vi "EOL NVH Outputs Controls Buffer 2.0.vi"(0 "Mode":T2, 1 "Motion Number":u16, 3 "Part Number":u16, 5 "NVH Outputs Control":T3[](array[typedef]), 7 "NVH Configuration":T1, 9 "NVH Outputs":bool[](array[boolean]), 11 "Serial Number In":string, 13 "ambient  temp (deg F)":dbl) -> (4 "NVH Outputs Out":bool[](array[boolean]), 6 "NVH Single Outputs":bool, 10 "Serial Number Out":string, 12 "NVH_PartNumber Out":u16, 14 "NVH_MotionNumber":u16, 15 "NVH All Outputs":bool[](array[boolean]))   [LabVIEW 2018]
uses:
  02.Type Def's/NVH Digital Output.ctl
  02.Type Def's/NVH Mode Control 2.0.ctl
  02.Type Def's/station nvh config.ctl
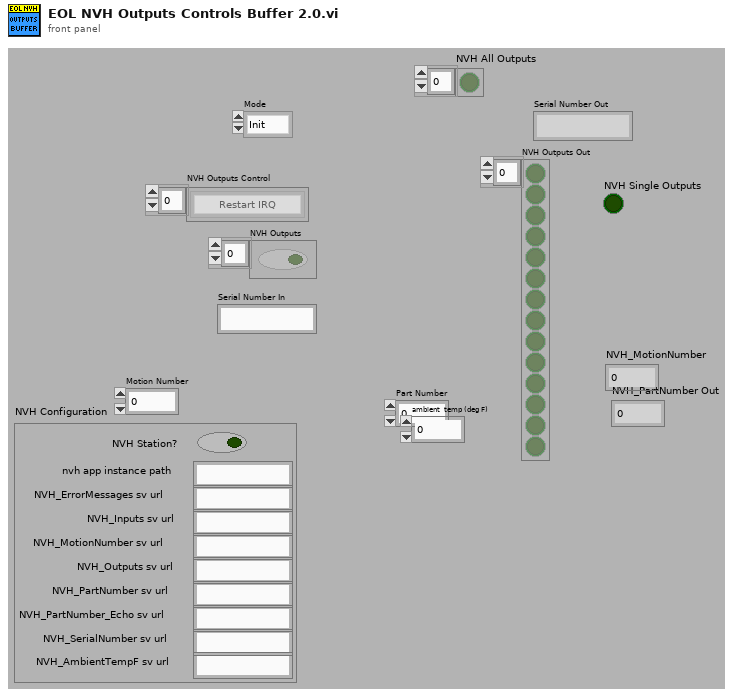
[diagram p1: front panel]
types:
  T1 = typedef "station nvh config.ctl" = cluster{"NVH Station?":bool, "nvh app instance path":string, "NVH_ErrorMessages sv url":string, "NVH_Inputs sv url":string, "NVH_MotionNumber sv url":string, "NVH_Outputs sv url":string, "NVH_PartNumber sv url":string, "NVH_PartNumber_Echo sv url":string, "NVH_SerialNumber sv url":string, "NVH_AmbientTempF sv url":string}
  T2 = typedef "NVH Mode Control 2.0.ctl" = enum16{"Init", "Write", "Write String", "Read", "Write Part Number", "Write Motion Number", "Write Ambient TempF"}
  T3 = typedef "NVH Digital Output.ctl" = enum16{"Restart IRQ", "Abort Test IRQ", "Read Model", "Start Test", "Stop Test", "End of Test IRQ", "Test Bit 1", "Test Bit 2", "Test Bit 3", "Test Bit 4", "Model Bit 1", "Model Bit 2", "Model Bit 3", "Model Bit 4", "Manual Restart IRQ"}
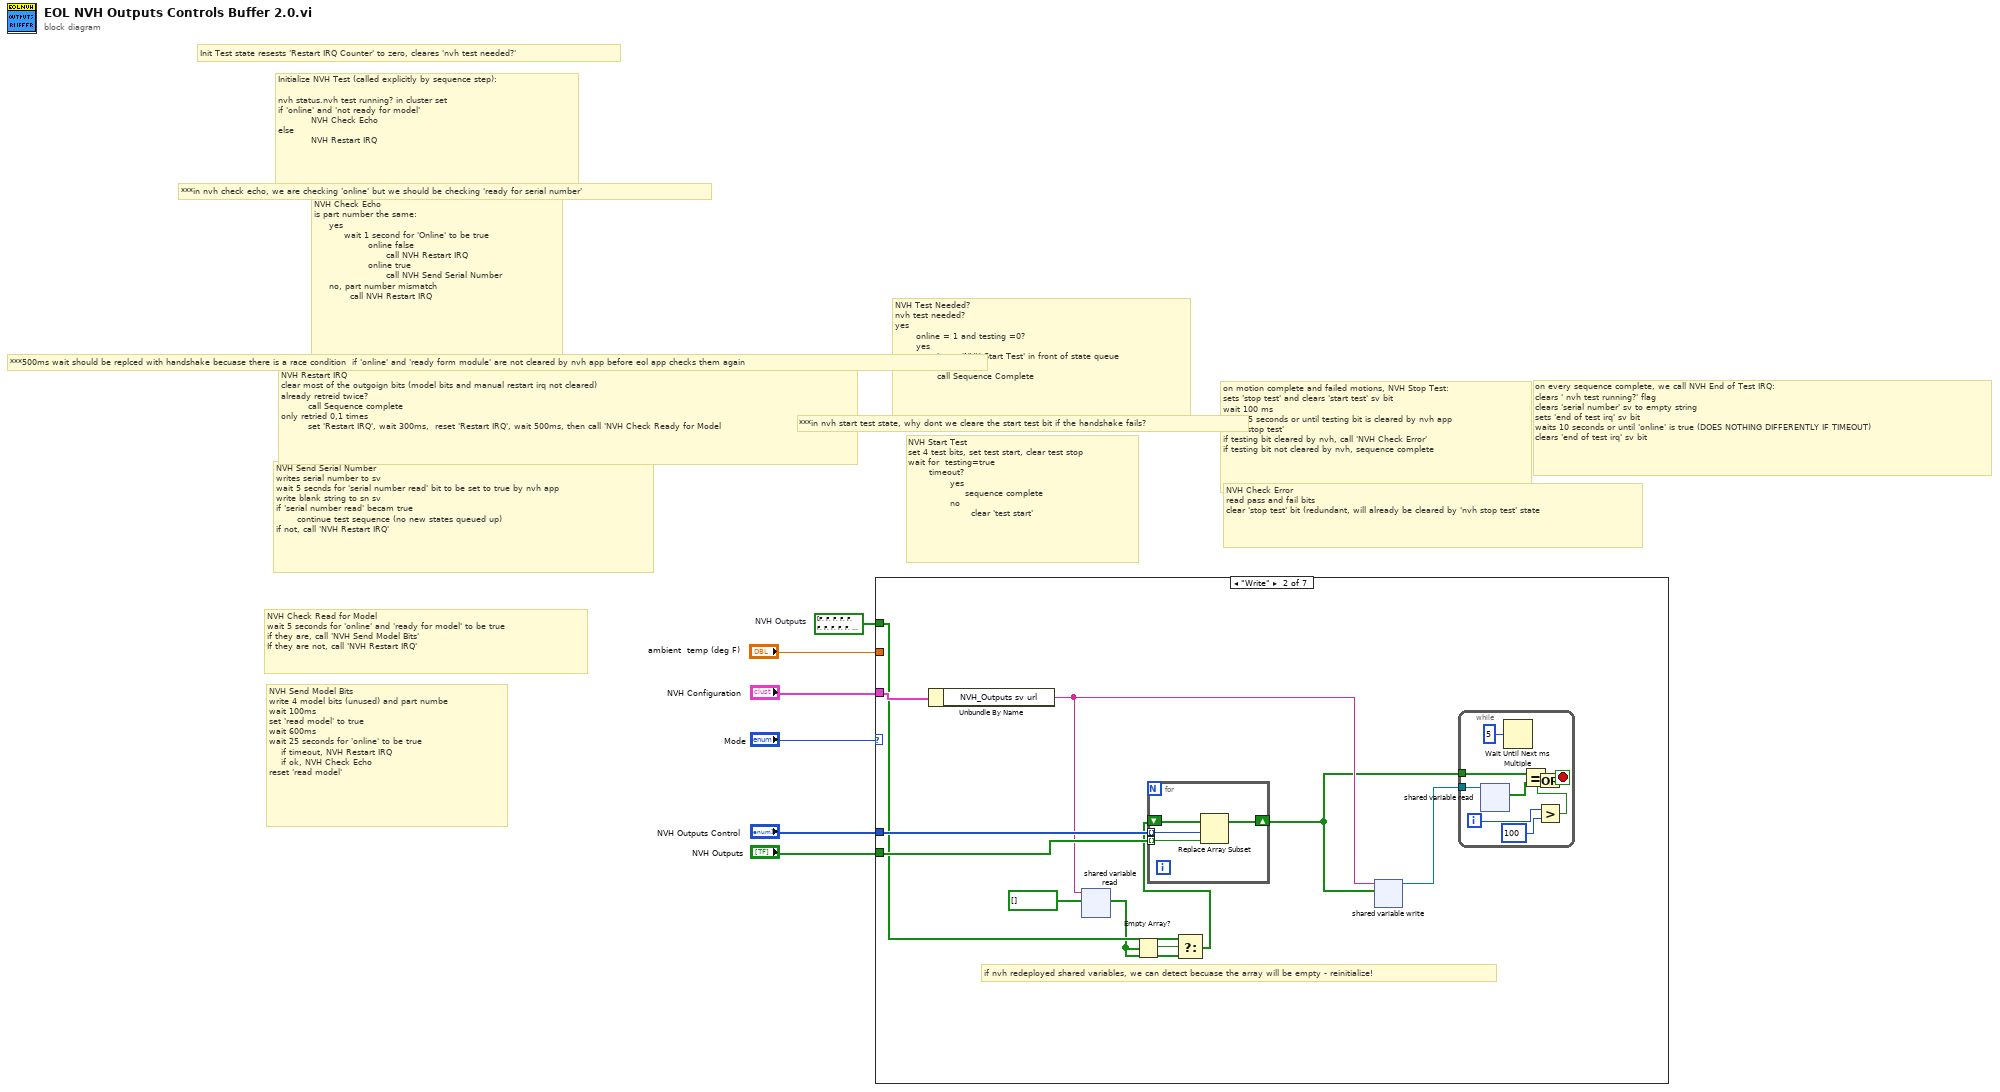
[diagram p0: block diagram]
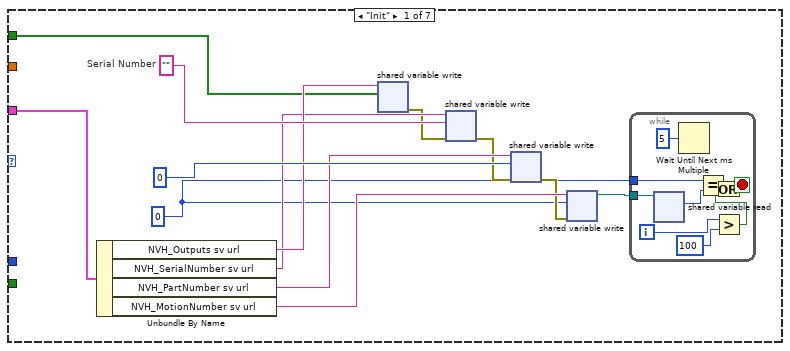
[diagram p2: hidden frame]
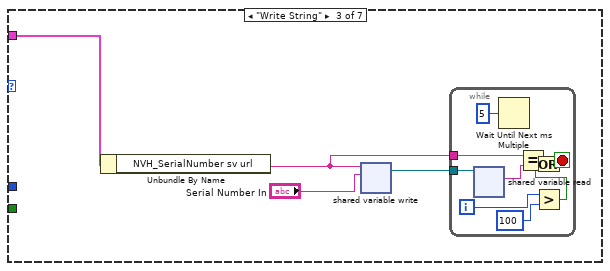
[diagram p3: hidden frame]
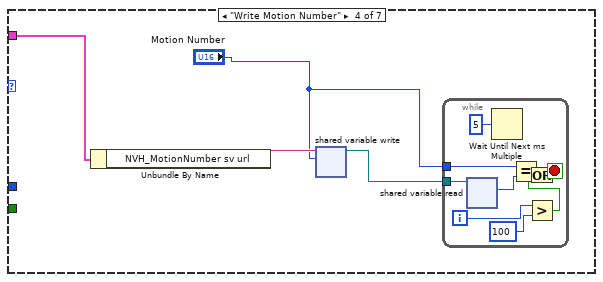
[diagram p4: hidden frame]
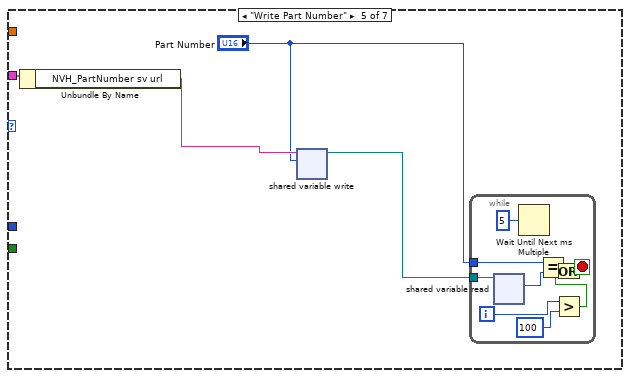
[diagram p5: hidden frame]
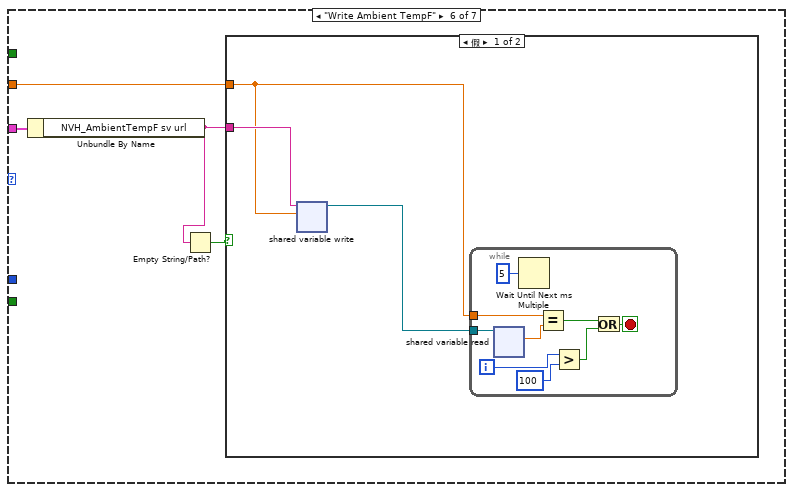
[diagram p6: hidden frame]
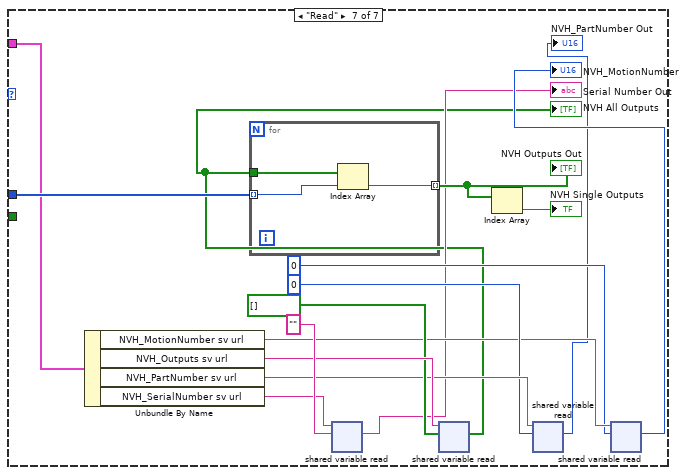
[diagram p8: hidden frame]
diagram:
  w2 = bool[] [FALSE, FALSE, FALSE, FALSE, FALSE, FALSE, FALSE, FALSE, FALSE, FALSE, FALSE, FALSE, FALSE, FALSE, FALSE]  # NVH Outputs
  # "NVH Check Error\nread pass and fail bits\nclear 'stop test' bit (redundant, will already be cleared by 'nvh stop test' state"
  # "NVH Send Model Bits\nwrite 4 model bits (unused) and part numbe\nwait 100ms\nset 'read model' to true\nwait 600ms\nwait 25 seconds for 'online' to be true\n    if timeout, NVH Restart IRQ\n    if ok, NVH Check Echo\nreset 'read model'"
  # "NVH Check Read for Model\nwait 5 seconds for 'online' and 'ready for model' to be true\nif they are, call 'NVH Send Model Bits'\nIf they are not, call 'NVH Restart IRQ'"
  # "***500ms wait should be replced with handshake becuase there is a race condition  if 'online' and 'ready form module' are not cleared by nvh app before eol app checks them again"
  # "Init Test state resests 'Restart IRQ Counter' to zero, cleares 'nvh test needed?'"
  # "NVH Send Serial Number\nwrites serial number to sv\nwait 5 secnds for 'serial number read' bit to be set to true by nvh app\nwrite blank string to sn sv\nif 'serial number read' becam true\n       continue test sequence (no new states queued up)\nif not, call 'NVH Restart IRQ'"
  # "NVH Restart IRQ\nclear most of the outgoign bits (model bits and manual restart irq not cleared)\nalready retreid twice?\n         call Sequence complete\nonly retried 0,1 times\n         set 'Restart IRQ', wait 300ms,  reset 'Restart IRQ', wait 500ms, then call 'NVH Check Ready for Model"
  # "***in nvh check echo, we are checking 'online' but we should be checking 'ready for serial number'"
  # "NVH Check Echo\nis part number the same:\n     yes\n          wait 1 second for 'Online' to be true\n                  online false\n                        call NVH Restart IRQ\n                  online true\n                        call NVH Send Serial Number\n     no, part number mismatch\n            call NVH Restart IRQ"
  # "Initialize NVH Test (called explicitly by sequence step):\n\nnvh status.nvh test running? in cluster set\nif 'online' and 'not ready for model'\n           NVH Check Echo\nelse\n           NVH Restart IRQ"
  # "on motion complete and failed motions, NVH Stop Test:\nsets 'stop test' and clears 'start test' sv bit\nwait 100 ms\nwait 15 seconds or until testing bit is cleared by nvh app\nclear 'stop test'\nif testing bit cleared by nvh, call 'NVH Check Error'\nif testing bit not cleared by nvh, sequence complete"
  # "on every sequence complete, we call NVH End of Test IRQ:\nclears ' nvh test running?' flag\nclears 'serial number' sv to empty string\nsets 'end of test irq' sv bit\nwaits 10 seconds or until 'online' is true (DOES NOTHING DIFFERENTLY IF TIMEOUT)\nclears 'end of test irq' sv bit"
  # "***in nvh start test state, why dont we cleare the start test bit if the handshake fails?"
  # "NVH Start Test\nset 4 test bits, set test start, clear test stop\nwait for  testing=true\n       timeout?\n              yes\n                   sequence complete\n              no\n                     clear 'test start'"
  # "NVH Test Needed?\nnvh test needed?\nyes\n       online = 1 and testing =0?\n       yes\n              insert 'NVH Start Test' in front of state queue\n       no\n              call Sequence Complete"
  n1 = case shown="\"Write\"" "Mode" {
    tunnel: "NVH Outputs Control" -> [_ w39 _ _ _ _ w123]
    tunnel: "NVH Outputs" -> [_ w38 _ _ _ _ _]
    tunnel: "NVH Configuration" -> [w17 w37 w55 w69 w82 w95 w113]
    tunnel: w2 -> [w7 w31 _ _ _ _ _]
    tunnel: "ambient  temp (deg F)" -> [_ _ _ _ _ w94 _]
    frame "Init" {
      w8 = u16 0 ("NVH_MotionNumber")
      w19 = ""  # Serial Number
      n2 = Unbundle By Name(w17) -> ("NVH_Outputs sv url"=w16:string, "NVH_SerialNumber sv url"=w15:string, "NVH_PartNumber sv url"=w14:string, "NVH_MotionNumber sv url"=w13:string)
      n3 = shared-variable-write(w16, w7) -> (w12:errorcluster)  [unwired: 1 in, 1 out]
      n4 = shared-variable-write(w15, w12, w19) -> (w11:errorcluster)  [unwired: 1 out]
      n5 = shared-variable-write(w14, w11, u16 0 ("NVH_PartNumber")) -> (w10:errorcluster)  [unwired: 1 out]
      n6 = shared-variable-write(w13, w10, w8) -> (w9:refnum<k21>)  [unwired: 1 out]
      n7 = while {
        tunnel: w9 -> [w28]
        tunnel: w8 -> [w25]
        i -> [w22]
        stop <- w23 stop-if-true
        n8 = shared-variable-read(w28) -> (w26:u16)  [unwired: 1 in, 3 out]
        n9 = Wait Until Next ms Multiple(millisecond multiple=u32 5) -> ()  [unwired: 1 out]
        n10 = Equal?(x=w25, y=w26) -> (x = y?=w24:bool)
        n11 = Greater?(x=w22, y=100) -> (0:w20:bool)
        n12 = Or(x=w24, y=w20) -> (x .or. y?=w23:bool)
      }
    }
    frame "Write" {
      # "if nvh redeployed shared variables, we can detect becuase the array will be empty - reinitialize!"
      n13 = Unbundle By Name(w37) -> ("NVH_Outputs sv url"=w35:string)
      n14 = shared-variable-read(w35, bool[] [] ("data out")) -> (w30:bool[])  [unwired: 1 in, 3 out]
      n15 = Empty Array?(array=w30) -> (empty?=w32:bool)
      n16 = Select(t=w31, s=w32, f=w30) -> (s? t:f=w29:bool[])
      n17 = for {
        shift-right: [w49] -> w34
        shift-left: w29 -> [w52]
        tunnel: w39 -> [w51] mode=indexing
        tunnel: w38 -> [w50] mode=indexing
        n18 = Replace Array Subset(array=w52, new element=w50, index=w51) -> (w49:bool[])
      }
      n19 = shared-variable-write(w35, w34) -> (w33:refnum<k21>)  [unwired: 1 in, 1 out]
      n20 = while {
        tunnel: w33 -> [w48]
        tunnel: w34 -> [w45]
        i -> [w42]
        stop <- w43 stop-if-true
        n21 = shared-variable-read(w48) -> (w46:bool[])  [unwired: 1 in, 3 out]
        n22 = Wait Until Next ms Multiple(millisecond multiple=u32 5) -> ()  [unwired: 1 out]
        n23 = Equal?(x=w45, y=w46) -> (x = y?=w44:bool)
        n24 = Greater?(x=w42, y=100) -> (0:w40:bool)
        n25 = Or(x=w44, y=w40) -> (x .or. y?=w43:bool)
      }
    }
    frame "Write String" {
      n26 = Unbundle By Name(w55) -> ("NVH_SerialNumber sv url"=w54:string)
      n27 = shared-variable-write(w54, "Serial Number In") -> (w53:refnum<k21>)  [unwired: 1 in, 1 out]
      n28 = while {
        tunnel: w53 -> [w65]
        tunnel: w54 -> [w62]
        i -> [w59]
        stop <- w60 stop-if-true
        n29 = shared-variable-read(w65) -> (w63:string)  [unwired: 1 in, 3 out]
        n30 = Wait Until Next ms Multiple(millisecond multiple=u32 5) -> ()  [unwired: 1 out]
        n31 = Equal?(x=w62, y=w63) -> (x = y?=w61:bool)
        n32 = Greater?(x=w59, y=100) -> (0:w57:bool)
        n33 = Or(x=w61, y=w57) -> (x .or. y?=w60:bool)
      }
    }
    frame "Write Motion Number" {
      n34 = Unbundle By Name(w69) -> ("NVH_MotionNumber sv url"=w68:string)
      n35 = shared-variable-write(w68, "Motion Number") -> (w66:refnum<k21>)  [unwired: 1 in, 1 out]
      n36 = while {
        tunnel: w66 -> [w78]
        tunnel: "Motion Number" -> [w75]
        i -> [w72]
        stop <- w73 stop-if-true
        n37 = shared-variable-read(w78) -> (w76:u16)  [unwired: 1 in, 3 out]
        n38 = Wait Until Next ms Multiple(millisecond multiple=u32 5) -> ()  [unwired: 1 out]
        n39 = Equal?(x=w75, y=w76) -> (x = y?=w74:bool)
        n40 = Greater?(x=w72, y=100) -> (0:w70:bool)
        n41 = Or(x=w74, y=w70) -> (x .or. y?=w73:bool)
      }
    }
    frame "Write Part Number" {
      n42 = Unbundle By Name(w82) -> ("NVH_PartNumber sv url"=w81:string)
      n43 = shared-variable-write(w81, "Part Number") -> (w80:refnum<k21>)  [unwired: 1 in, 1 out]
      n44 = while {
        tunnel: w80 -> [w91]
        tunnel: "Part Number" -> [w88]
        i -> [w85]
        stop <- w86 stop-if-true
        n45 = shared-variable-read(w91) -> (w89:u16)  [unwired: 1 in, 3 out]
        n46 = Wait Until Next ms Multiple(millisecond multiple=u32 5) -> ()  [unwired: 1 out]
        n47 = Equal?(x=w88, y=w89) -> (x = y?=w87:bool)
        n48 = Greater?(x=w85, y=100) -> (0:w83:bool)
        n49 = Or(x=w87, y=w83) -> (x .or. y?=w86:bool)
      }
    }
    frame "Write Ambient TempF" {
      n50 = Unbundle By Name(w95) -> ("NVH_AmbientTempF sv url"=w93:string)
      n51 = Empty String/Path?(string/path=w93) -> (empty?=w92:bool)
      n52 = case shown="假" w92 {
        tunnel: w93 -> [w98 _]
        tunnel: w94 -> [w96 _]
        frame False {
          n53 = shared-variable-write(w98, w96) -> (w97:refnum<k21>)  [unwired: 1 in, 1 out]
          n54 = while {
            tunnel: w97 -> [w107]
            tunnel: w96 -> [w104]
            i -> [w101]
            stop <- w102 stop-if-true
            n55 = shared-variable-read(w107) -> (w105:dbl)  [unwired: 1 in, 3 out]
            n56 = Wait Until Next ms Multiple(millisecond multiple=u32 5) -> ()  [unwired: 1 out]
            n57 = Equal?(x=w104, y=w105) -> (x = y?=w103:bool)
            n58 = Greater?(x=w101, y=100) -> (0:w99:bool)
            n59 = Or(x=w103, y=w99) -> (x .or. y?=w102:bool)
          }
        }
        frame True {
        }
      }
    }
    frame "Read" {
      n60 = Unbundle By Name(w113) -> ("NVH_MotionNumber sv url"=w115:string, "NVH_Outputs sv url"=w119:string, "NVH_PartNumber sv url"=w117:string, "NVH_SerialNumber sv url"=w110:string)
      n61 = shared-variable-read(w110, "" ("Serial Number Out")) -> (→"Serial Number Out":string)  [unwired: 1 in, 3 out]
      n62 = shared-variable-read(w119, bool[] [] ("data out")) -> (w108:bool[])  [unwired: 1 in, 3 out]
      "NVH All Outputs" <- w108
      n63 = for {
        tunnel: w123 -> [w125] mode=indexing
        tunnel: w108 -> [w126]
        tunnel: [w124] -> w122 mode=indexing
        n64 = Index Array(array=w126, index=w125) -> (element=w124:bool)
      }
      "NVH Outputs Out" <- w122
      n65 = Index Array(array=w122) -> (element=→"NVH Single Outputs":bool)  [unwired: 1 in]
      n66 = shared-variable-read(w117, u16 0 ("data out")) -> (→"NVH_PartNumber Out":u16)  [unwired: 1 in, 3 out]
      n67 = shared-variable-read(w115, u16 0 ("NVH_MotionNumber Out")) -> (→"NVH_MotionNumber":u16)  [unwired: 1 in, 3 out]
    }
  }
